vi "PMU_CFG-2_PACK.vi"(1 "String":string) -> (0 "PMU1 CFG Packet":string[](array[string]))   [LabVIEW 2013]
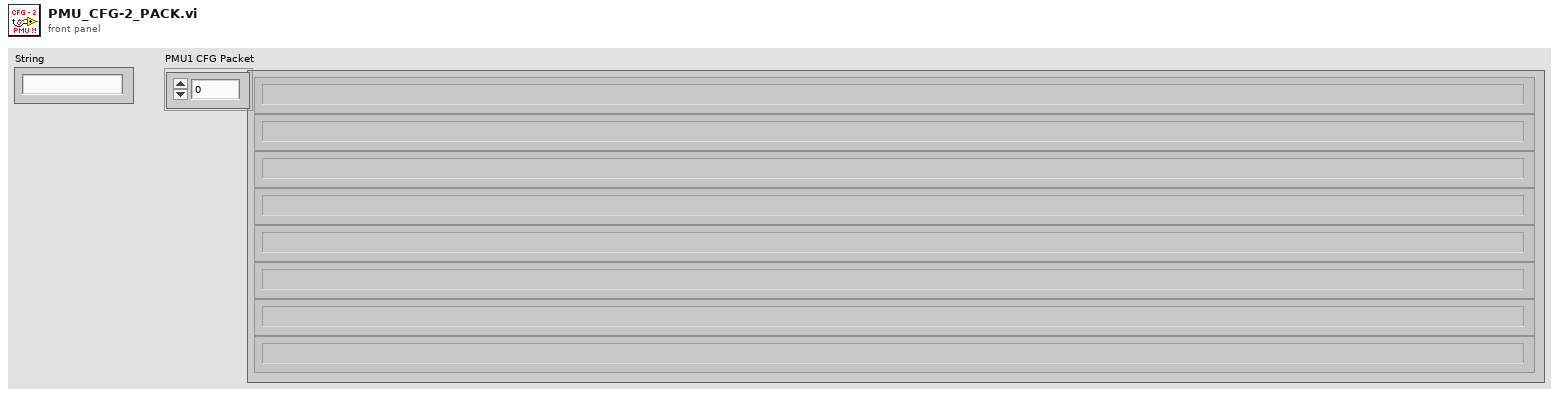
[diagram p1: front panel]
types:
  T1 = cluster{"SYNC":u32, "FRAMSIZE":u32, "IDCODE":u32, "SOC":u64, "DATA_RATE":u32, "FRACSEC":u64, "TIME_BASE":u32, "NUM_PMU":u32}
  T2 = cluster{"PHNUMR":u16, "ANNUMR":u16, "DGNUMR":u16}
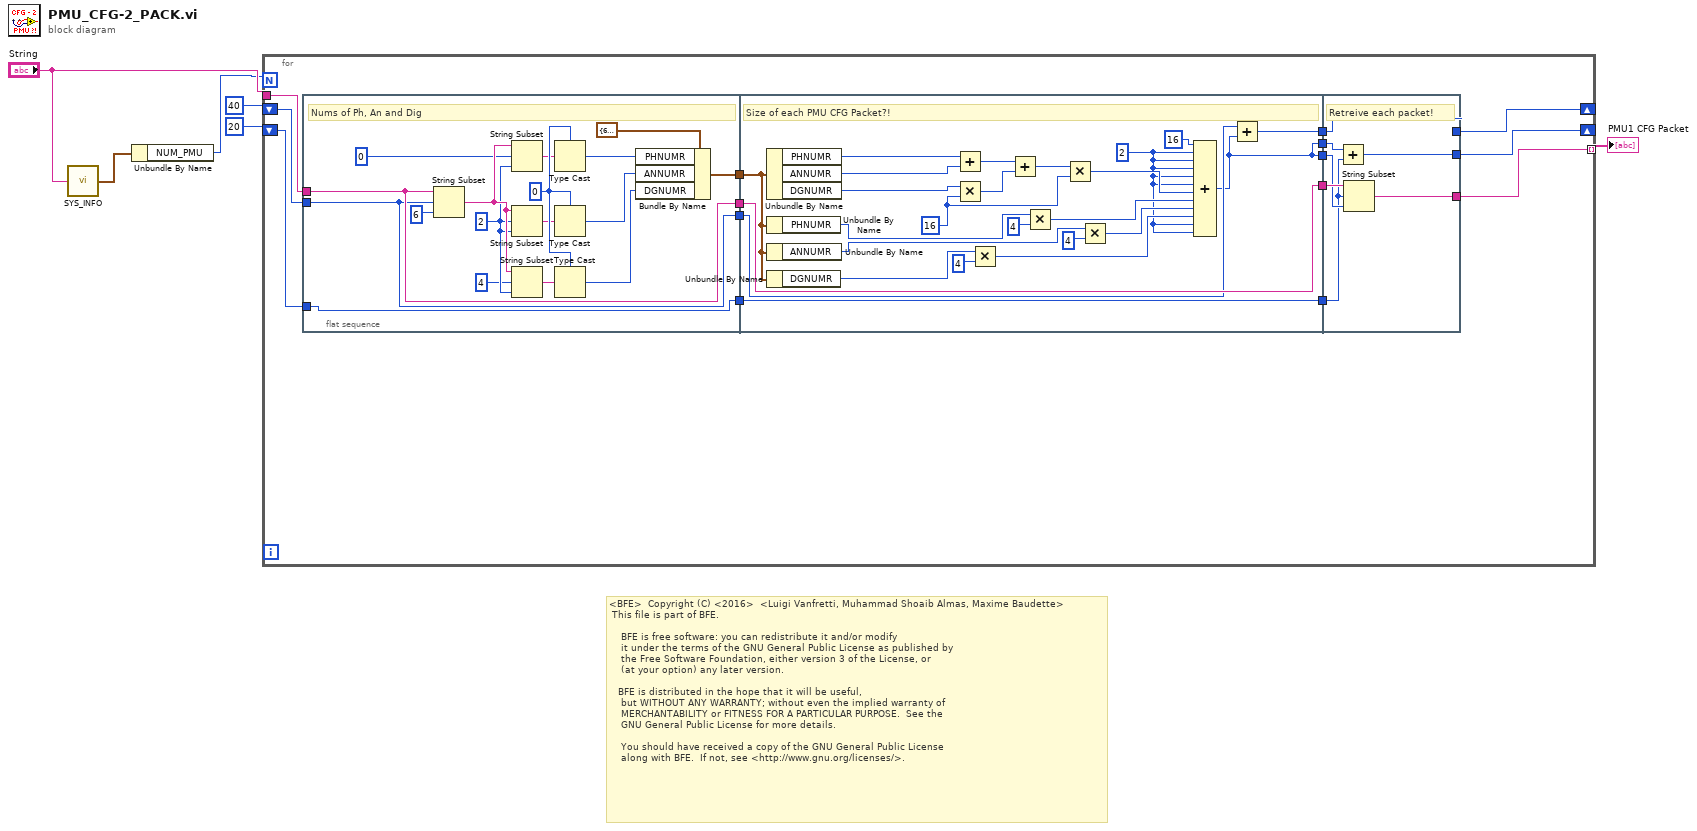
[diagram p0: block diagram]
diagram:
  # "<BFE>  Copyright (C) <2016>  <Luigi Vanfretti, Muhammad Shoaib Almas, Maxime Baudette>\n This file is part of BFE.\n\n    BFE is free software: you can redistribute it and/or modify\n    it under the terms of the GNU General Public License as published by\n    the Free Software Foundation, either version 3 of the License, or\n    (at your option) any later version.\n\n   BFE is distributed in the hope that it will be useful,\n    but WITHOUT ANY WARRANTY; without even the implied warranty of\n    MERCHANTABILITY or FITNESS FOR A PARTICULAR PURPOSE.  See the\n    GNU General Public License for more details.\n\n    You should have received a copy of the GNU General Public License\n    along with BFE.  If not, see <http://www.gnu.org/licenses/>."
  n1 = call "SYS_INFO.vi"("CFG-2"="String") -> ("output cluster"=w6:T1)
  n2 = Unbundle By Name(w6) -> ("NUM_PMU"=w2:u32)
  n3 = for {
    N: w2 -> [_]
    tunnel: "String" -> [w21]
    shift-right: [w9] -> _
    shift-left: 40 -> [w20]
    shift-right: [w12] -> _
    shift-left: 20 -> [w13]
    tunnel: [w11] -> w4 mode=indexing
    n4 = flat-sequence {
      tunnel: w21 -> [w24]
      tunnel: w20 -> [w22]
      tunnel: [w25] -> w19
      tunnel: [w24] -> w17
      tunnel: [w23] -> w14
      tunnel: w13 -> [w23]
      tunnel: [w22] -> w8
      tunnel: w19 -> [w46]
      tunnel: [w43] -> w18
      tunnel: w17 -> [w43]
      tunnel: [w39] -> w16
      tunnel: [w42] -> w15
      tunnel: w14 -> [w42]
      tunnel: [w41] -> w10
      tunnel: w8 -> [w40]
      tunnel: [w39] -> w7
      tunnel: w18 -> [w70]
      tunnel: w16 -> [w69]
      tunnel: w15 -> [w65]
      tunnel: [w64] -> w12
      tunnel: [w68] -> w11
      tunnel: w10 -> [w67]
      tunnel: [w67] -> w9
      tunnel: w7 -> [w66]
      frame #0 {
        w33 = u16 0
        w35 = 2 ("length (rest)")
        # "Nums of Ph, An and Dig"
        n5 = String Subset(string=w24, offset (0)=w22, length (rest)=6 ("length (rest)")) -> (substring=w38:string)
        n6 = String Subset(string=w38, offset (0)=0, length (rest)=w35) -> (substring=w32:string)
        n7 = String Subset(string=w38, offset (0)=w35, length (rest)=w35) -> (substring=w31:string)
        n8 = String Subset(string=w38, offset (0)=4, length (rest)=w35) -> (substring=w30:string)
        n9 = Type Cast(type=w33, x=w32) -> (*(type *) &x=w29:u16)
        n10 = Type Cast(type=w33, x=w31) -> (*(type *) &x=w28:u16)
        n11 = Type Cast(type=w33, x=w30) -> (*(type *) &x=w27:u16)
        n12 = Bundle By Name(cluster=T2 {"PHNUMR"=6, "ANNUMR"=3, "DGNUMR"=1}, "PHNUMR"=w29, "ANNUMR"=w28, "DGNUMR"=w27) -> (w25:T2)
      }
      frame #1 {
        w56 = u16 16 ("y")
        w44 = u8 2 ("value")
        # "Size of each PMU CFG Packet?!"
        n13 = Unbundle By Name(w46) -> ("PHNUMR"=w62:u16, "ANNUMR"=w61:u16, "DGNUMR"=w60:u16)
        n14 = Unbundle By Name(w46) -> ("PHNUMR"=w54:u16)
        n15 = Unbundle By Name(w46) -> ("ANNUMR"=w50:u16)
        n16 = Unbundle By Name(w46) -> ("DGNUMR"=w48:u16)
        n17 = Add(x=w62, y=w61) -> (x+y=w58:u16)
        n18 = Multiply(x=w60, y=w56) -> (x*y=w59:u16)
        n19 = Multiply(x=w48, y=u16 4) -> (x*y=w45:u16)
        n20 = Add(x=w58, y=w59) -> (x+y=w57:u16)
        n21 = Multiply(x=w54, y=u16 4) -> (x*y=w52:u16)
        n22 = Multiply(x=w57, y=w56) -> (x*y=w55:u16)
        n23 = Multiply(x=w50, y=u16 4) -> (x*y=w49:u16)
        n24 = Compound Arithmetic op=ADD(u8 16 ("value"), w44, w44, w44, w44, w44, w55, w52, w49, w45, w44, w44) -> (w39:u16)
        n25 = Add(x=w40, y=w39) -> (x+y=w41:i32)
      }
      frame #2 {
        # "Retreive each packet!"
        n26 = Add(x=w66, y=w65) -> (x+y=w64:i32)
        n27 = String Subset(string=w70, offset (0)=w65, length (rest)=w69) -> (substring=w68:string)
      }
    }
  }
  "PMU1 CFG Packet" <- w4
